vi "Mixer.IsAvailable.vi"(0 "address":string) -> (1 "available":bool, 2 "message":string)   [LabVIEW 2020]
uses:
  <vilib>/httpClient/LabVIEWHTTPClient.lvlib
panel:
  out "body":string
  out "headers":string
  out "error out":errorcluster
  in  "error in (no error)":errorcluster
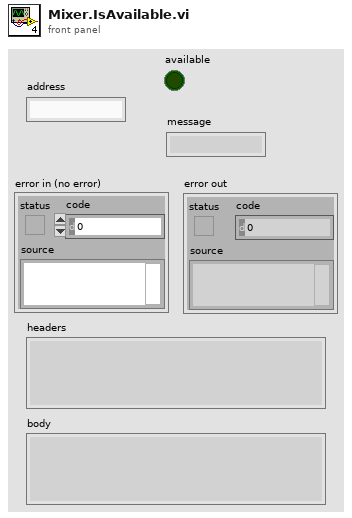
[diagram p1: front panel]
types:
  T1 = typedef "LabVIEWHTTPClient.lvlib/ClientHandle.ctl" = refnum<k1>
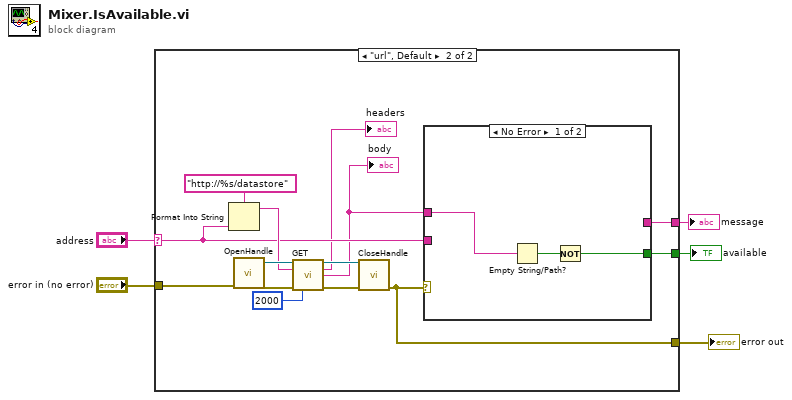
[diagram p0: block diagram]
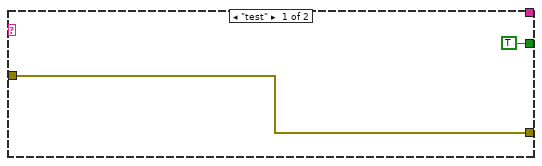
[diagram p2: hidden frame]
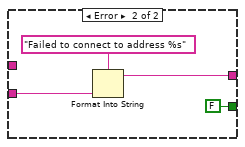
[diagram p3: hidden frame]
diagram:
  n1 = case shown="\"url\", Default" "address" {
    selector: "address" -> [_ w14]
    tunnel: "error in (no error)" -> [w6 w18]
    tunnel: [_ w13] -> w3
    tunnel: [TRUE w12] -> w2
    tunnel: [w6 w8] -> w1
    frame "test" {
    }
    frame "url", Default {
      n2 = Format Into String(format string="http://%s/datastore", w14) -> (resulting string=w15:string)  [unwired: 2 in, 1 out]
      n3 = call <vilib>:"OpenHandle.vi"("error in (no error)"=w18) -> ("client handle out"=w21:T1, "error out"=w19:errorcluster)  [unwired: 13 in]
      n4 = call <vilib>:"GET.vi"("client handle"=w21, "url"=w15, "error in (no error)"=w19, "timeout (10000)"=2000) -> ("client handle out"=w20:T1, "headers"=→"headers":string, "body"=w9:string, "error out"=w17:errorcluster)  [unwired: 8 in]
      "body" <- w9
      n5 = call <vilib>:"CloseHandle.vi"("client handle"=w20, "error in (no error)"=w17) -> ("error out"=w8:errorcluster)  [unwired: 13 in]
      n6 = case shown="No Error" w8 {
        tunnel: w14 -> [_ w28]
        tunnel: [_ w26] -> w13
        tunnel: [w22 FALSE] -> w12
        tunnel: w9 -> [w24 _]
        frame No Error {
          n7 = Empty String/Path?(string/path=w24) -> (empty?=w23:bool)
          n8 = Not(x=w23) -> (.not. x?=w22:bool)
        }
        frame Error {
          n9 = Format Into String(format string="Failed to connect to address %s" ("Message"), w28) -> (resulting string=w26:string)  [unwired: 2 in, 1 out]
        }
      }
    }
  }
  "available" <- w2
  "message" <- w3
  "error out" <- w1
